vi "Sample Array To Waveforms.vi"(8 "sample_rate":u32, 9 "channels":u32, 10 "num_samples":u64, 11 "sample_data":i16[](array[numeric])) -> (3 "Waveform Data":waveform(i16)[](array[waveform]))   [LabVIEW 2020, in "G-Audio.lvlib"]
doc: "Decimates sample_data according to the number of channels, and places the decimated array into a waveform. Each waveform corresponds to a channel of data."
uses:
  G-Audio.lvlib
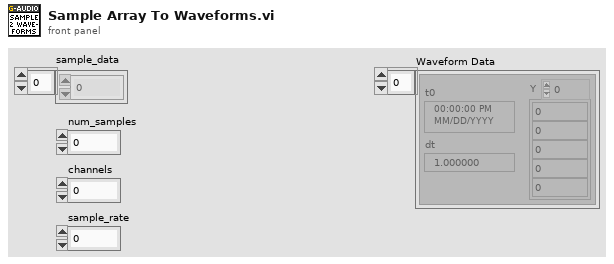
[diagram p1: front panel]
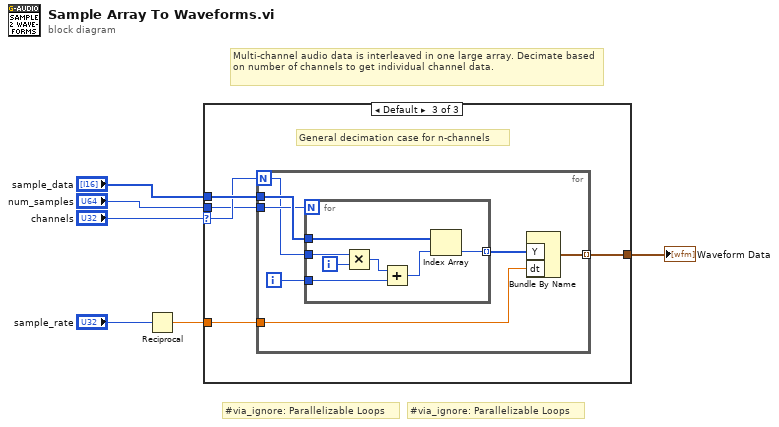
[diagram p0: block diagram]
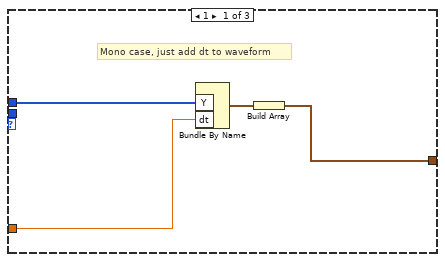
[diagram p2: hidden frame]
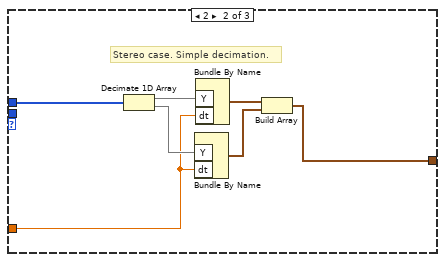
[diagram p3: hidden frame]
diagram:
  # "Multi-channel audio data is interleaved in one large array. Decimate based on number of channels to get individual channel data."
  # "#via_ignore: Parallelizable Loops"
  # "#via_ignore: Parallelizable Loops"
  n1 = Reciprocal(x="sample_rate") -> (1/x=w5:dbl)
  n2 = case shown="Default" "channels" {
    selector: "channels" -> [_ _ w19]
    tunnel: "sample_data" -> [w10 w15 w22]
    tunnel: [w7 w16 w21] -> w1
    tunnel: w5 -> [w9 w12 w20]
    tunnel: "num_samples" -> [_ _ w18]
    frame 1 {
      # "Mono case, just add dt to waveform"
      n3 = Bundle By Name("Y"=w10, "dt"=w9) -> (w8:waveform(i16))  [unwired: 1 in]
      n4 = Build Array(w8) -> (w7:waveform(i16)[])
    }
    frame 2 {
      # "Stereo case. Simple decimation."
      n5 = Decimate 1D Array(w15) -> (w14:i16[], w13:i16[])
      n6 = Bundle By Name("Y"=w13, "dt"=w12) -> (w11:waveform(i16))  [unwired: 1 in]
      n7 = Bundle By Name("Y"=w14, "dt"=w12) -> (w17:waveform(i16))  [unwired: 1 in]
      n8 = Build Array(w17, w11) -> (w16:waveform(i16)[])
    }
    frame Default {
      # "General decimation case for n-channels"
      n9 = for {
        N: w19 -> [w23]
        tunnel: w22 -> [w29]
        tunnel: w18 -> [w28]
        tunnel: [w26] -> w21 mode=indexing
        tunnel: w20 -> [w25]
        i -> [w27]
        n10 = for {
          N: w28 -> [_]
          tunnel: w29 -> [w36]
          tunnel: w27 -> [w34]
          tunnel: [w31] -> w24 mode=indexing
          tunnel: w23 -> [w30]
          i -> [w35]
          n11 = Multiply(x=w30, y=w35) -> (x*y=w33:i32)
          n12 = Add(x=w33, y=w34) -> (x+y=w32:i32)
          n13 = Index Array(array=w36, index=w32) -> (element=w31:i16)
        }
        n14 = Bundle By Name("Y"=w24, "dt"=w25) -> (w26:waveform(i16))  [unwired: 1 in]
      }
    }
  }
  "Waveform Data" <- w1
